vi "Xtarget.vi"(8 "error in (no error)":errorcluster, 9 "Controls":i32[](array[numeric]), 10 "Target in":T1, 11 "Gate in":refnum<class "G-UE.lvclass">) -> (0 "error out":errorcluster, 2 "Target out":T1, 3 "Gate out":refnum<class "G-UE.lvclass">)   [LabVIEW 2016, in "G-UE.lvclass"]
uses:
  G-UE.lvclass
  TypeDefs/Circuit Cluster.ctl
  GateAbst/GateAbst.lvclass
  G-UE.lvclass/G-UE.ctl
  <vilib>/Analysis/baseanly.llb/Complex A x B.vi
  <vilib>/Analysis/NI_AALBase.lvlib
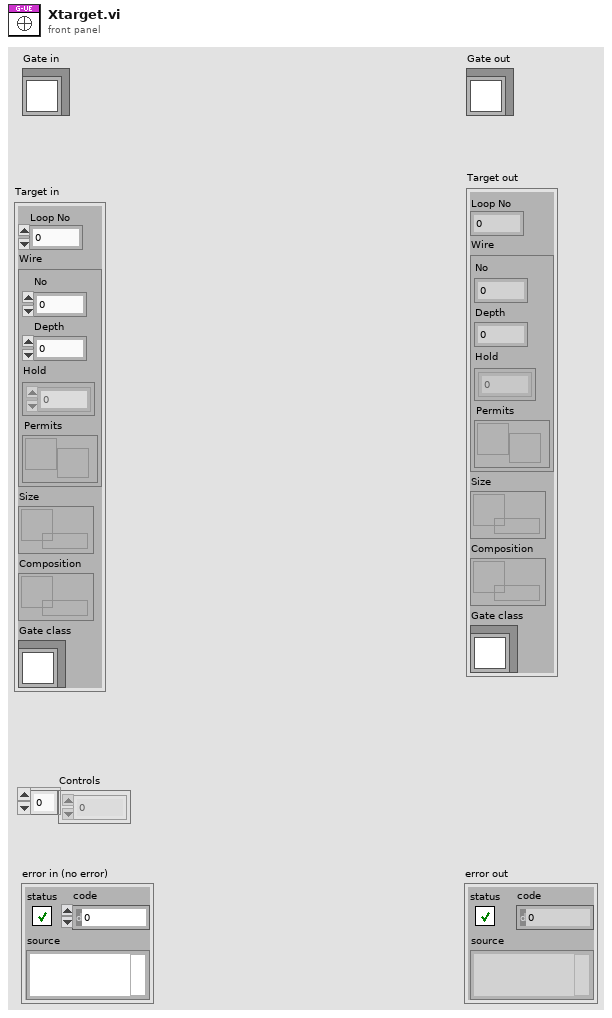
[diagram p1: front panel]
types:
  T1 = typedef "Circuit Cluster.ctl" = cluster{"Loop No":i32, "Wire":cluster{"No":i32, "Depth":i32, "Hold":i32[][], "Permits":refnum<notifier>}, "Size":refnum<queue>, "Composition":refnum<queue>, "Gate class":refnum<class "GateAbst.lvclass">}
  T2 = typedef "NI_Matrix.lvlib/ComplexMatrix.ctl" = cdb[][]
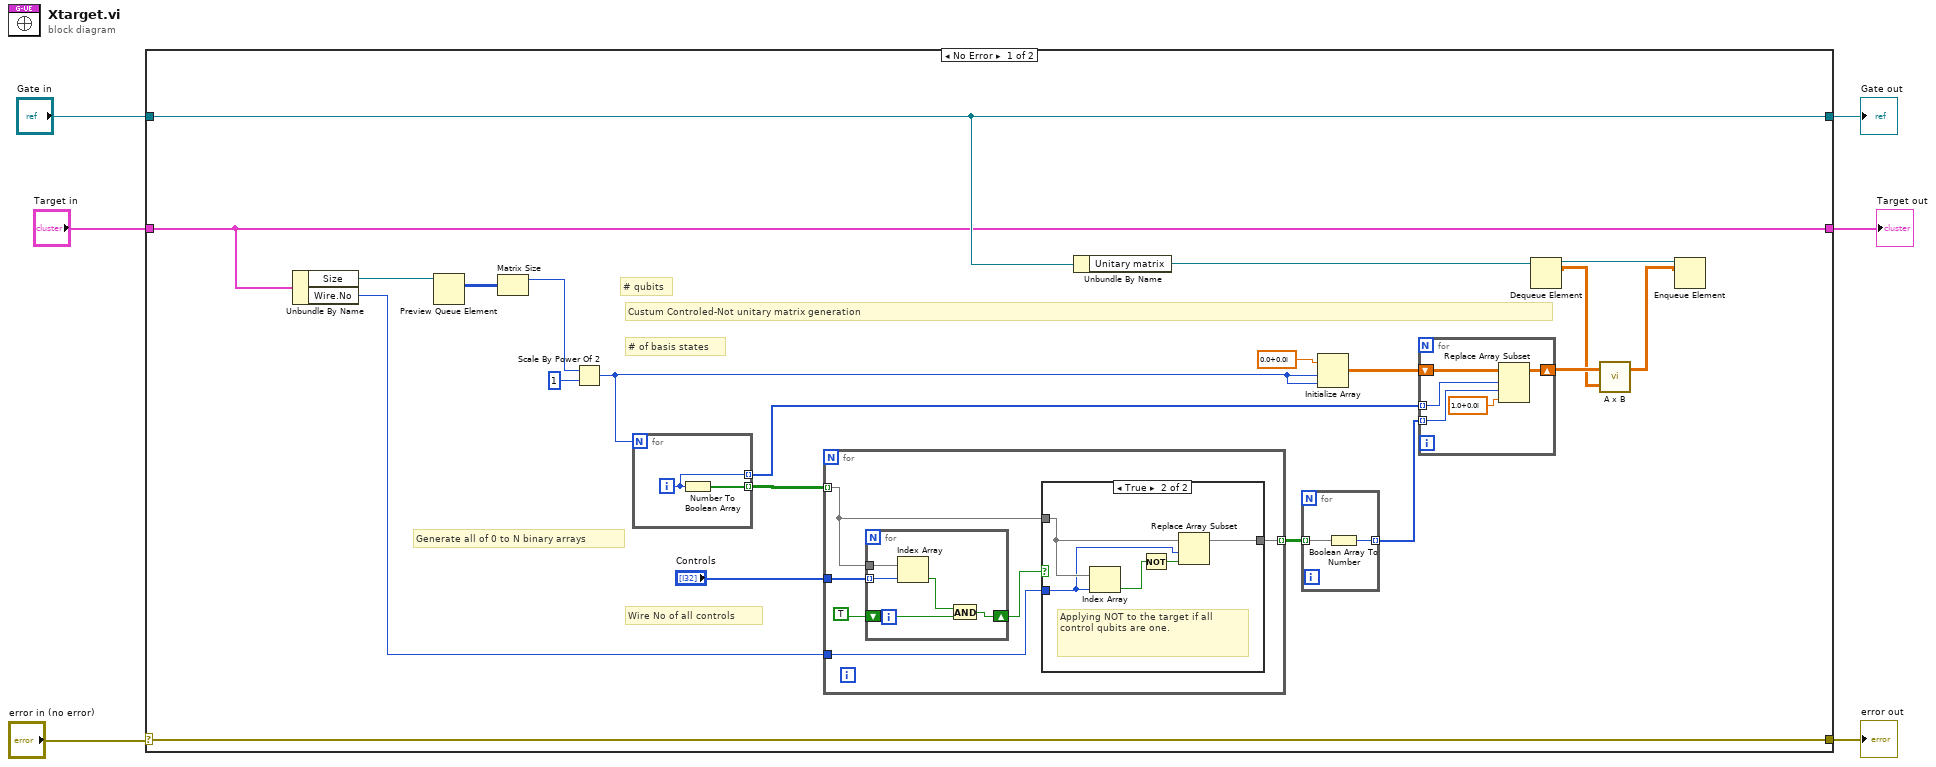
[diagram p0: block diagram]
diagram:
  n1 = case shown="No Error" "error in (no error)" {
    selector: "error in (no error)" -> [w27 w56]
    tunnel: [w27 w56] -> w5
    tunnel: [w17 w55] -> w3
    tunnel: "Gate in" -> [w17 w55]
    tunnel: "Target in" -> [w9 w54]
    tunnel: [w9 w54] -> w1
    frame No Error {
      # "Custum Controled-Not unitary matrix generation"
      # "Wire No of all controls"
      # "# of basis states"
      # "# qubits"
      # "Generate all of 0 to N binary arrays"
      n2 = Unbundle By Name(w9) -> ("Size"=w12:refnum<queue>, "Wire.No"=w18:i32)
      n3 = Preview Queue Element(queue=w12) -> (element=w8:i32[][])  [unwired: 2 in, 3 out]
      n4 = Matrix Size(0:w8) -> (1:w7:i32)  [unwired: 1 out]
      n5 = Scale By Power Of 2(n=w7, x=1) -> (x*2^n=w10:i32)
      n6 = for {
        N: w10 -> [_]
        tunnel: [w29] -> w21 mode=indexing
        tunnel: [w28] -> w25 mode=indexing
        i -> [w28]
        n7 = Number To Boolean Array(number=w28) -> (Boolean array=w29:bool[])
      }
      n8 = for {
        tunnel: w21 -> [w33] mode=indexing
        tunnel: w18 -> [w34]
        tunnel: [w35] -> w22 mode=indexing
        tunnel: "Controls" -> [w32]
        n9 = for {
          tunnel: w33 -> [w39]
          tunnel: w32 -> [w36] mode=indexing
          shift-right: [w37] -> w30
          shift-left: TRUE -> [w38]
          n10 = Index Array "Index Array"(array=w39, index=w36) -> (element=w40:bool)
          n11 = And(x=w40, y=w38) -> (x .and. y?=w37:bool)
        }
        n12 = case shown="True" w30 {
          tunnel: w33 -> [w41 w46]
          tunnel: w34 -> [_ w44]
          tunnel: [w41 w42] -> w35
          frame False {
          }
          frame True {
            # "Applying NOT to the target if all control qubits are one."
            n13 = Index Array(array=w46, index=w44) -> (element=w45:bool)
            n14 = Not(x=w45) -> (.not. x?=w43:bool)
            n15 = Replace Array Subset(array=w46, new element=w43, index=w44) -> (w42:bool[])
          }
        }
      }
      n16 = Unbundle By Name(w17) -> ("Unitary matrix"=w15:refnum<queue>)
      n17 = for {
        tunnel: w22 -> [w53] mode=indexing
        tunnel: [w52] -> w24 mode=indexing
        n18 = Boolean Array To Number(Boolean array=w53) -> (number=w52:u32)
      }
      n19 = Initialize Array "Initialize Array"(cdb 0.0+0.0i ("element"), w10, w10) -> (w26:cdb[][])
      n20 = for {
        tunnel: w24 -> [w49] mode=indexing
        tunnel: w25 -> [w48] mode=indexing
        shift-right: [w47] -> w19
        shift-left: w26 -> [w51]
        n21 = Replace Array Subset(array=w51, new element=cdb 1.0+0.0i ("new element/subarray"), index (row)=w48, index (col)=w49) -> (w47:cdb[][])
      }
      n22 = Dequeue Element(queue=w15) -> (queue out=w13:refnum<queue>, element=w14:T2)  [unwired: 2 in, 2 out]
      n23 = call-poly <vilib>:"A x B.vi"("B"=w14, "A"=w19) -> ("A x B"=w16:T2)  [unwired: 1 out]
      n24 = Enqueue Element(queue=w13, element=w16) -> ()  [unwired: 2 in, 3 out]
    }
    frame Error {
    }
  }
  "error out" <- w5
  "Gate out" <- w3
  "Target out" <- w1
